vi "Split Logs.vi"(8 "error in (no error)":errorcluster, 11 "Historian Logger in":refnum<class "Historian Logger.lvclass">) -> (0 "error out":errorcluster, 3 "Historian Logger out":refnum<class "Historian Logger.lvclass">)   [LabVIEW 2020, in "VolatusHistorian.lvlib" / "Historian Logger.lvclass"]
uses:
  Historian Logger.lvclass
  Historian Logger.lvclass/Historian Logger.ctl
  Volatus/MessageQ/MessageQ.lvclass
  VolatusErrorUtilities/MultiErrors/MultiErrors.lvclass
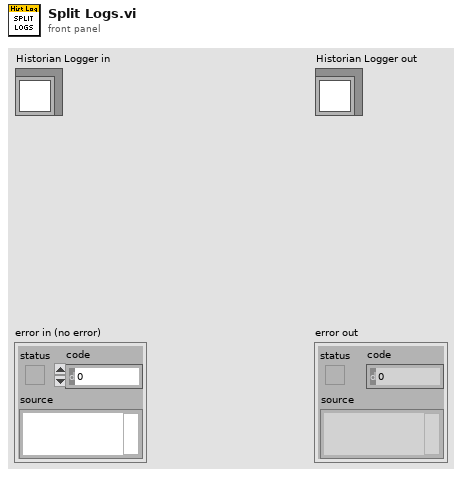
[diagram p1: front panel]
types:
  T1 = typedef "VolatusHistorian.lvlib/Historian Logger.lvclass/Group Info.ctl" = cluster{"Buffer":refnum<class "Group Buffer DBL.lvclass">, "Logger":refnum<class "MessageQ.lvclass">, "Group":refnum<class "Group.lvclass">, "Last Timestamp":dbl, "State":T2}
  T2 = typedef "VolatusData.lvlib/Logger State.ctl" = enum16{"Unknown", "Idle", "Preparing", "Ready", "Logging", "Stopping"}
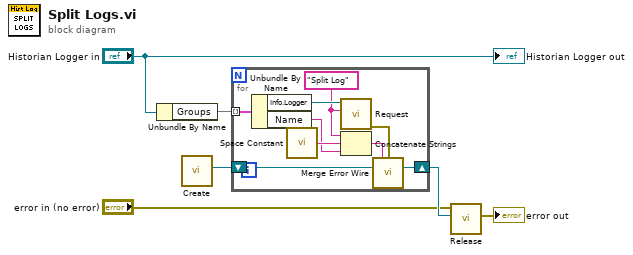
[diagram p0: block diagram]
diagram:
  n1 = Unbundle By Name("Historian Logger in") -> ("Groups"=w5:map{string, T1})
  n2 = call "Create.vi"() -> ("MultiErrors out"=w4:refnum<class "MultiErrors.lvclass">)  [unwired: 11 in]
  n3 = for {
    tunnel: w5 -> [w15] mode=indexing
    shift-right: [w12] -> w3
    shift-left: w4 -> [w13]
    w8 = "Split Log" ("ID")
    n4 = Unbundle By Name(w15) -> ("Info.Logger"=w14:refnum<class "MessageQ.lvclass">, "Name"=w9:string)
    n5 = call <vilib>:"Space Constant.vi"() -> ("String"=w10:string)
    n6 = call "Request.vi"("ID"=w8, "MessageQ in"=w14) -> ("error out"=w11:errorcluster)  [unwired: 7 in, 2 out]
    n7 = Concatenate Strings(w8, w10, w9) -> (w7:string)
    n8 = call "Merge Error Wire.vi"("Local Context (None)"=w7, "error in (no error)"=w11, "MultiErrors in"=w13) -> ("MultiErrors out"=w12:refnum<class "MultiErrors.lvclass">)  [unwired: 12 in]
  }
  n9 = call "Release.vi"("MultiErrors in"=w3, "Upstream Error (None)"="error in (no error)") -> ("error out"=→"error out":errorcluster)  [unwired: 9 in]
  "Historian Logger out" <- "Historian Logger in"
